vi "Printer Comm Handler.vi"(1 "Printer Comm CMDs":T1) -> ()   [LabVIEW 2021]
uses:
  C:/Users/enProducts/Downloads/KIA_Enproducts/KIA_Enproducts/Global VIs/Controls/Device Generic Comm CMDs.ctl
  C:/Users/enProducts/Downloads/KIA_Enproducts/KIA_Enproducts/Global VIs/Controls/Device Generic Commands.ctl
  C:/Users/enProducts/Downloads/KIA_Enproducts/KIA_Enproducts/Global VIs/Controls/Genric Q Action.ctl
  Device Manager/Printer/Sub VIs/Zebra Printer/Zebra_Printer/Zebra_Printer.lvclass
panel:
  in  "Printer CMD":string
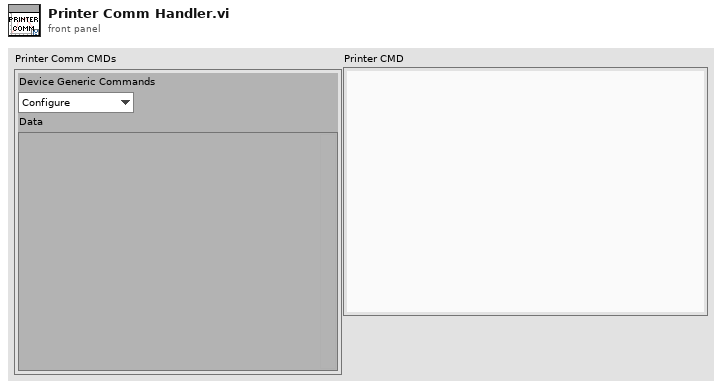
[diagram p1: front panel]
types:
  T1 = typedef "Device Generic Comm CMDs.ctl" = cluster{"Device Generic Commands":T2, "Data":variant}
  T2 = typedef "Device Generic Commands.ctl" = enum16{"Configure", "Connect", "Write", "Read", "Write and Read", "Write and Read Specific Msg", "DUT App SW Flash", "Flush Input Buffer", "Disconnect", "Start Tester", "Stop Tester", "Write Tester Channel", ""}
  T3 = typedef "Genric Q Action.ctl" = enum16{"Create", "Enqueue", "Dequeue", "Flush", "Clear"}
  T4 = enum16{"Yet to Configure", "Configured", "Connected", "Disconnected", "Error"}
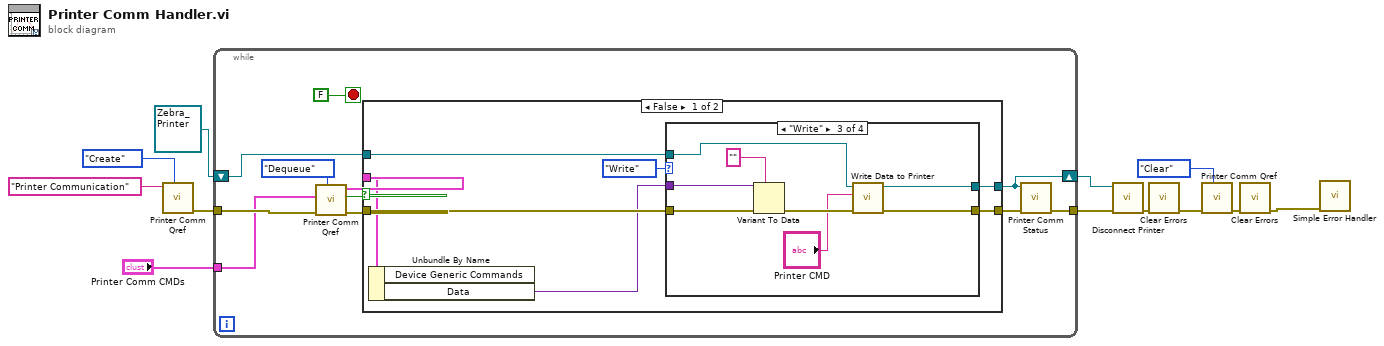
[diagram p0: block diagram]
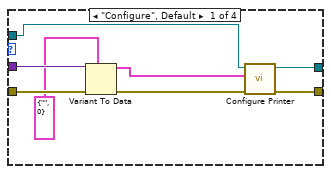
[diagram p2: hidden frame]
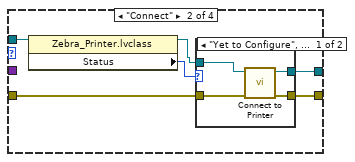
[diagram p3: hidden frame]
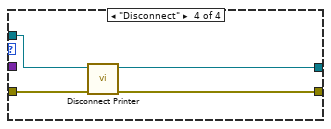
[diagram p5: hidden frame]
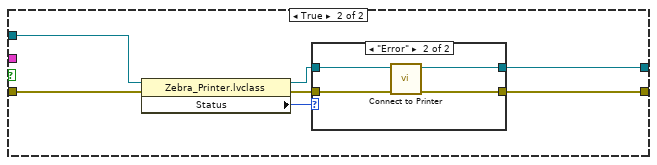
[diagram p6: hidden frame]
diagram:
  n1 = call "Printer Comm Qref.vi"("Generic Q Action"=Genric_Q_Action."Create", "Q Name"="Printer Communication") -> ("error out"=w7:errorcluster)  [unwired: 7 in, 2 out]
  n2 = while {
    tunnel: w7 -> [w22]
    shift-right: [w16] -> w6
    shift-left: refnum<class "Zebra_Printer.lvclass"> refnum ("Zebra_Printer.lvclass") -> [w19]
    tunnel: [w14] -> w2
    tunnel: "Printer Comm CMDs" -> [w13]
    stop <- FALSE stop-if-true
    n3 = call "Printer Comm Qref.vi"("Generic Q Action"=Genric_Q_Action."Dequeue", "error in (no error)"=w22, "Printer Comm CMDs"=w13) -> ("error out"=w18:errorcluster, "timed out?"=w21:bool, "DUT Comm CMDs"=w20:T1)  [unwired: 6 in]
    n4 = case shown="False" w21 {
      tunnel: w20 -> [w30 _]
      tunnel: w19 -> [w29 w69]
      tunnel: [w28 w67] -> w16
      tunnel: w18 -> [w27 w65]
      tunnel: [w26 w63] -> w17
      frame False {
        n5 = Unbundle By Name(w30) -> ("Data"=w25:variant)  [unwired: 1 out]
        n6 = case shown="\"Write\"" Device_Generic_Commands."Write" ("Device Generic Commands") {
          tunnel: w29 -> [w36 w44 w58 w62]
          tunnel: [w35 w43 w54 w61] -> w28
          tunnel: w27 -> [w37 w42 w56 w60]
          tunnel: [w33 w41 w53 w59] -> w26
          tunnel: w25 -> [w38 _ w57 _]
          frame "Configure", Default {
            n7 = Variant To Data(error in=w37, type=cluster{"IP Adress":string, "Port":i16} {"IP Adress"="", "Port"=0} ("Printer Configuration"), Variant=w38) -> (data=w31:cluster{"IP Adress":string, "Port":i16}, error out=w34:errorcluster)
            n8 = call-dynamic "Configure Printer.vi"("error in (no error)"=w34, "Printer Configuration"=w31, "Zebra_Printer in"=w36) -> ("error out"=w33:errorcluster, "Zebra_Printer out"=w35:refnum<class "Zebra_Printer.lvclass">)  [unwired: 7 in]
          }
          frame "Connect" {
            n9 = property class="Zebra_Printer.lvclass"(reference=w44) -> (reference out=w40:refnum<class "Zebra_Printer.lvclass">, "Status"=w39:T4)  [unwired: 1 in, 1 out]
            n10 = case shown="\"Yet to Configure\", Default" w39 {
              tunnel: w40 -> [w48 w49]
              tunnel: [w47 w49] -> w43
              tunnel: w42 -> [w46 w50]
              tunnel: [w45 w50] -> w41
              frame "Yet to Configure", Default {
                n11 = call-dynamic "Connect to Printer.vi"("error in (no error)"=w46, "Zebra_Printer in"=w48) -> ("error out"=w45:errorcluster, "Zebra_Printer out"=w47:refnum<class "Zebra_Printer.lvclass">)  [unwired: 8 in]
              }
              frame "Connected" {
              }
            }
          }
          frame "Write" {
            n12 = Variant To Data(error in=w56, type="", Variant=w57) -> (error out=w55:errorcluster)  [unwired: 1 out]
            n13 = call-dynamic "Write Data to Printer.vi"("error in"=w55, "Printer CMD"="Printer CMD", "Zebra_Printer in"=w58) -> ("error out"=w53:errorcluster, "Zebra_Printer out"=w54:refnum<class "Zebra_Printer.lvclass">)  [unwired: 7 in]
          }
          frame "Disconnect" {
            n14 = call-dynamic "Disconnect Printer.vi"("error in"=w60, "Zebra_Printer in"=w62) -> ("error out"=w59:errorcluster, "Zebra_Printer out"=w61:refnum<class "Zebra_Printer.lvclass">)  [unwired: 8 in]
          }
        }
      }
      frame True {
        n15 = property class="Zebra_Printer.lvclass"(reference=w69, error in=w65) -> (reference out=w66:refnum<class "Zebra_Printer.lvclass">, error out=w64:errorcluster, "Status"=w68:T4)
        n16 = case shown="\"Error\"" w68 {
          tunnel: [w70 w73] -> w67
          tunnel: w66 -> [w70 w75]
          tunnel: w64 -> [w71 w74]
          tunnel: [w71 w72] -> w63
          frame "Yet to Configure", Default {
          }
          frame "Error" {
            n17 = call-dynamic "Connect to Printer.vi"("error in (no error)"=w74, "Zebra_Printer in"=w75) -> ("error out"=w72:errorcluster, "Zebra_Printer out"=w73:refnum<class "Zebra_Printer.lvclass">)  [unwired: 8 in]
          }
        }
      }
    }
    n18 = call "Printer Comm Status.vi"("error in (no error)"=w17, "Zebra_Printer.lvclass"=w16) -> ("error out"=w14:errorcluster)  [unwired: 9 in]
  }
  n19 = call-dynamic "Disconnect Printer.vi"("error in"=w2, "Zebra_Printer in"=w6) -> ("error out"=w5:errorcluster)  [unwired: 8 in, 1 out]
  n20 = call <vilib>:"Clear Errors.vi"("error in (no error)"=w5) -> ("error out"=w4:errorcluster)  [unwired: 5 in, 1 out]
  n21 = call "Printer Comm Qref.vi"("Generic Q Action"=Genric_Q_Action."Clear", "error in (no error)"=w4) -> ("error out"=w10:errorcluster)  [unwired: 7 in, 2 out]
  n22 = call <vilib>:"Clear Errors.vi"("error in (no error)"=w10) -> ("error out"=w3:errorcluster)  [unwired: 5 in, 1 out]
  n23 = call <vilib>:"Simple Error Handler.vi"("error in (no error)"=w3) -> ()  [unwired: 4 in, 5 out]
